vi "mukodo.vi"() -> ()   [LabVIEW 2016]
uses:
  <vilib>/Instr/_visa.llb/VISA Configure Serial Port (Instr).vi
panel:
  in  "Lock":bool
  in  "Slide":u8(slide) scale=0.0..90.0
  out "?":i32
  out "Waveform Chart":i32(graph)
  out "Available?":bool
  in  "COM Port":refnum<visa-resource-name>
  in  "Stop Button":bool
  in  "Auto":bool
  in  "Manual":bool
  # "ARDUINO"
  # "USB Control"
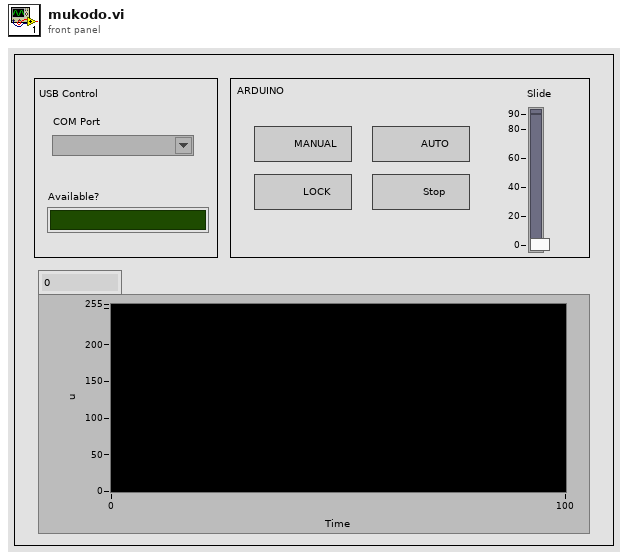
[diagram p1: front panel]
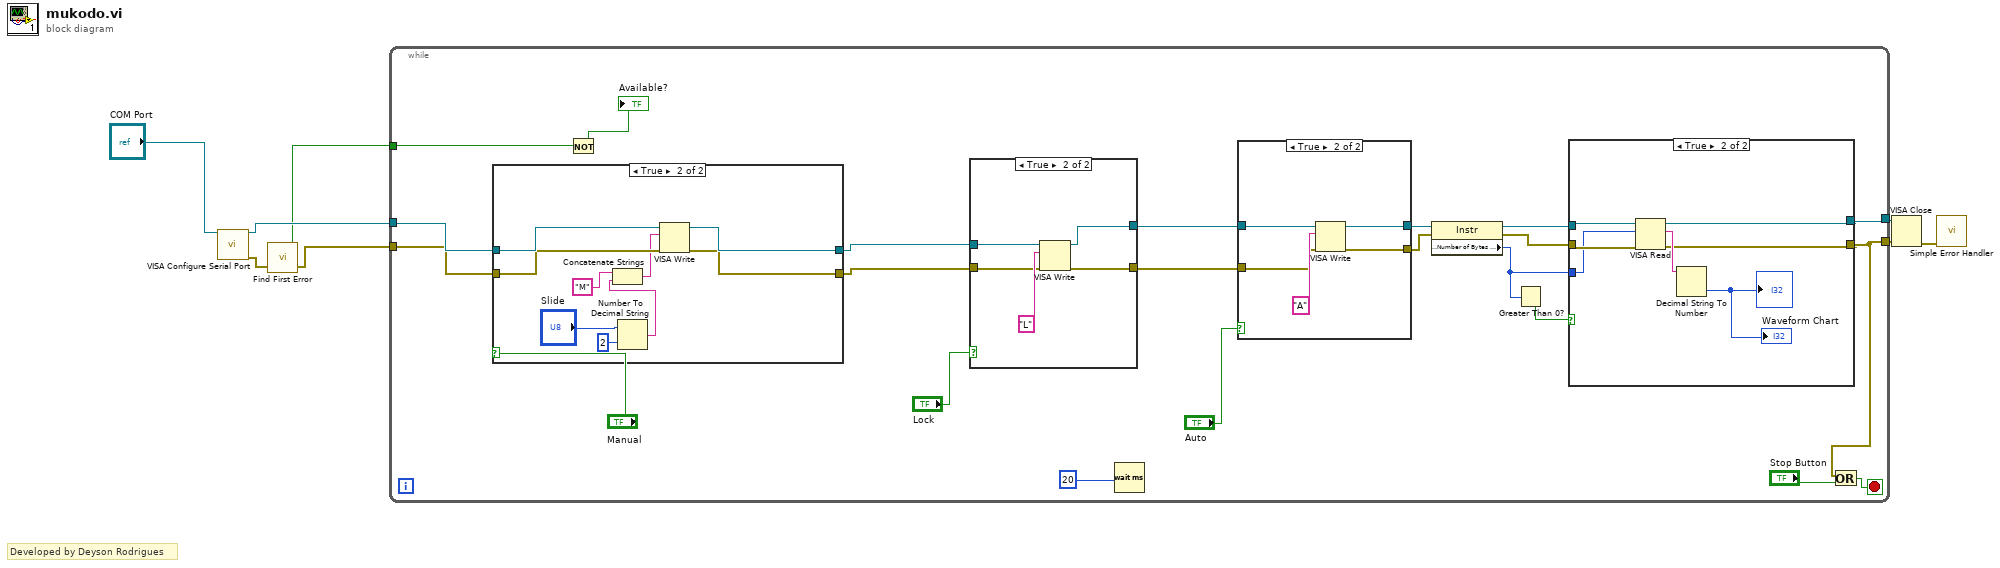
[diagram p0: block diagram]
diagram:
  # "Developed by Deyson Rodrigues"
  n1 = call-poly "VISA Configure Serial Port"("VISA resource name"="COM Port") -> ("VISA resource name out"=w3:refnum<visa-resource-name>, "error out"=w5:errorcluster)  [unwired: 13 in]
  n2 = call <vilib>:"Find First Error.vi"("error in (no error)"=w5) -> ("error out"=w2:errorcluster, "error?"=w1:bool)  [unwired: 3 in]
  n3 = while {
    tunnel: [w25] -> w7
    tunnel: [w14] -> w8
    tunnel: w3 -> [w19]
    tunnel: w2 -> [w18]
    tunnel: w1 -> [w17]
    stop <- w15 stop-if-true
    n4 = case shown="True" "Manual" {
      tunnel: [w55 w64] -> w12
      tunnel: [w54 w63] -> w11
      tunnel: w19 -> [w55 w62]
      tunnel: w18 -> [w54 w61]
      frame False {
      }
      frame True {
        n5 = Number To Decimal String(number="Slide", width (-)=i16 2) -> (decimal integer string=w58:string)
        n6 = Concatenate Strings("M" ("write buffer"), w58) -> (w57:string)
        n7 = VISA Write(VISA resource name=w62, write buffer=w57, error in (no error)=w61) -> (VISA resource name out=w64:refnum<visa-resource-name>, error out=w63:errorcluster)  [unwired: 1 out]
      }
    }
    n8 = Not(x=w17) -> (.not. x?=→"Available?":bool)
    n9 = case shown="True" "Lock" {
      tunnel: w12 -> [w32 w36]
      tunnel: w11 -> [w31 w35]
      tunnel: [w32 w34] -> w10
      tunnel: [w31 w33] -> w9
      frame False {
      }
      frame True {
        n10 = VISA Write(VISA resource name=w36, write buffer="L", error in (no error)=w35) -> (VISA resource name out=w34:refnum<visa-resource-name>, error out=w33:errorcluster)  [unwired: 1 out]
      }
    }
    n11 = Wait (ms)(milliseconds to wait=u32 20 ("millisecond timer value")) -> ()  [unwired: 1 out]
    n12 = case shown="True" "Auto" {
      tunnel: [w47 w53] -> w29
      tunnel: [w48 w52] -> w30
      tunnel: w10 -> [w48 w50]
      tunnel: w9 -> [w47 w49]
      frame False {
      }
      frame True {
        n13 = VISA Write(VISA resource name=w50, write buffer="A", error in (no error)=w49) -> (VISA resource name out=w52:refnum<visa-resource-name>, error out=w53:errorcluster)  [unwired: 1 out]
      }
    }
    n14 = property class="Instr"(reference=w30, error in=w29) -> (reference out=w26:refnum<visa-resource-name>, error out=w27:errorcluster, "Serial Settings:Number of Bytes at Serial Port"=w24:u32)
    n15 = Greater Than 0?(x=w24) -> (x > 0?=w28:bool)
    n16 = case shown="True" w28 {
      tunnel: w26 -> [w39 w43]
      tunnel: w27 -> [w38 w44]
      tunnel: [w39 w41] -> w25
      tunnel: [w38 w40] -> w14
      tunnel: w24 -> [_ w42]
      frame False {
      }
      frame True {
        n17 = VISA Read(VISA resource name=w43, byte count=w42, error in (no error)=w44) -> (VISA resource name out=w41:refnum<visa-resource-name>, read buffer=w46:string, error out=w40:errorcluster)  [unwired: 1 out]
        n18 = Decimal String To Number(string=w46) -> (number=→"Waveform Chart" →"?":i32)  [unwired: 2 in, 1 out]
      }
    }
    n19 = Or(x=w14, y="Stop Button") -> (x .or. y?=w15:bool)
  }
  n20 = VISA Close(VISA resource name=w7, error in (no error)=w8) -> (error out=w6:errorcluster)
  n21 = call <vilib>:"Simple Error Handler.vi"("error in (no error)"=w6) -> ()  [unwired: 4 in, 5 out]
